vi "Aquire Image.vi"(4 "error out":errorcluster, 5 "Last Buffer aquired":i32, 6 "New Image":T1, 7 "IMAQ Session Out 2":refnum<k11>) -> (0 "error out":errorcluster, 1 "Image Out":T1, 2 "Buffer Index Copied":i32, 3 "IMAQ Session Out":refnum<k11>)   [LabVIEW 2009]
uses:
  <vilib>/vision/Image Controls.llb/IMAQ Image.ctl
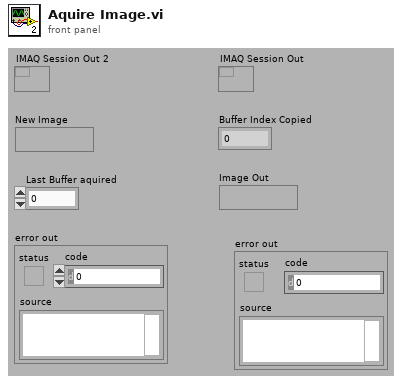
[diagram p1: front panel]
types:
  T1 = typedef "IMAQ Image.ctl" = refnum<image>
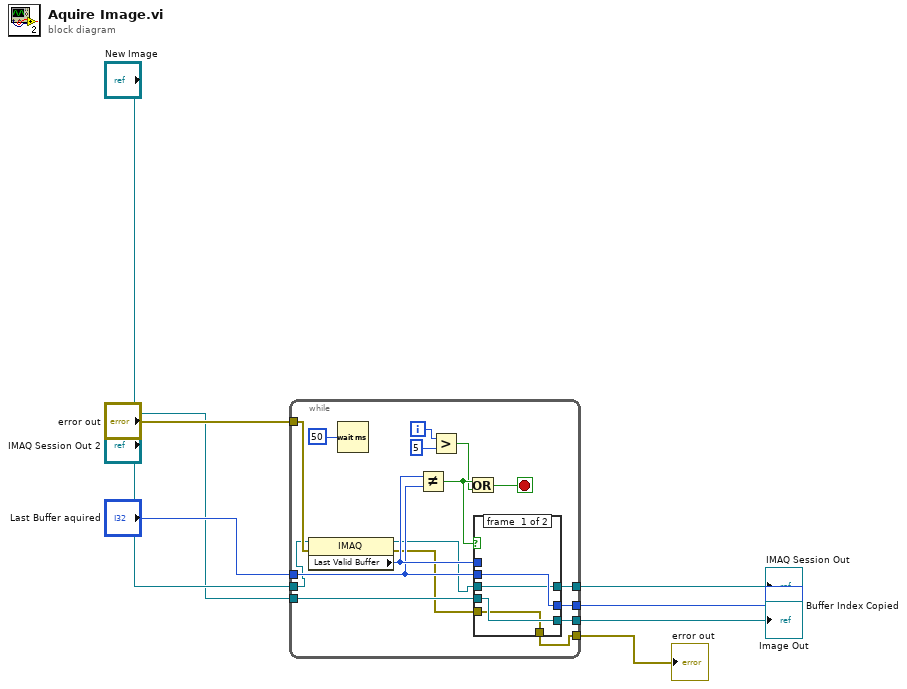
[diagram p0: block diagram]
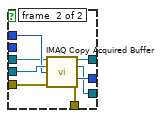
[diagram p2: hidden frame]
diagram:
  n1 = while {
    tunnel: [w24] -> w7
    tunnel: "Last Buffer aquired" -> [w21]
    tunnel: "New Image" -> [w23]
    tunnel: "IMAQ Session Out 2" -> [w10]
    tunnel: [w15] -> w6
    tunnel: [w14] -> w8
    tunnel: "error out" -> [w13]
    tunnel: [w11] -> w1
    i -> [w20]
    stop <- w16 stop-if-true
    n2 = property class="IMAQ"(reference=w10, error in=w13) -> (reference out=w9:refnum<k11>, error out=w12:errorcluster, "Last Valid Buffer"=w22:u32)
    n3 = Wait (ms)(milliseconds to wait=u32 50) -> ()  [unwired: 1 out]
    n4 = Not Equal?(x=w22, y=w21) -> (x != y?=w18:bool)
    n5 = Greater?(x=w20, y=5) -> (0:w17:bool)
    n6 = Or(x=w18, y=w17) -> (x .or. y?=w16:bool)
    n7 = case shown="True" w18 {
      tunnel: [w29 w37] -> w24
      tunnel: w23 -> [w27 w36]
      tunnel: w22 -> [_ w35]
      tunnel: w21 -> [w29 _]
      tunnel: w9 -> [w28 w34]
      tunnel: [w28 w33] -> w15
      tunnel: [w27 w32] -> w14
      tunnel: w12 -> [w26 w31]
      tunnel: [w26 w30] -> w11
      frame #0 {
      }
      frame #1 {
        n8 = call <vilib>:"IMAQ Copy Acquired Buffer.vi"("IMAQ Session In"=w34, "Image In"=w36, "Buffer Number"=w35, "error in (no error)"=w31) -> ("IMAQ Session Out"=w33:refnum<k11>, "Image Out"=w32:T1, "Buffer Index Copied"=w37:i32, "error out"=w30:errorcluster)  [unwired: 7 in, 1 out]
      }
    }
  }
  "Image Out" <- w8
  "Buffer Index Copied" <- w7
  "IMAQ Session Out" <- w6
  "error out" <- w1
